vi "FGV_Stop_Error.vi"(7 "Action":enum16{"Read", "Write"}(ring), 8 "Error In (no error)":errorcluster, 10 "Var In":bool) -> (0 "Error Out":errorcluster, 2 "Var Out":bool)   [LabVIEW 2018]
doc: "FGV for stop loop value."
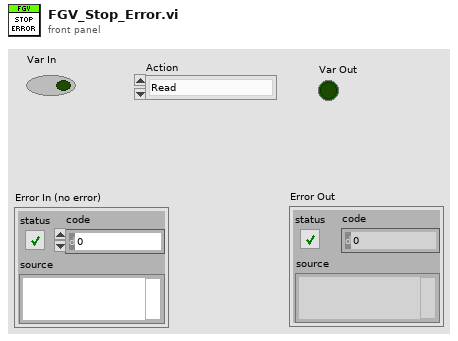
[diagram p1: front panel]
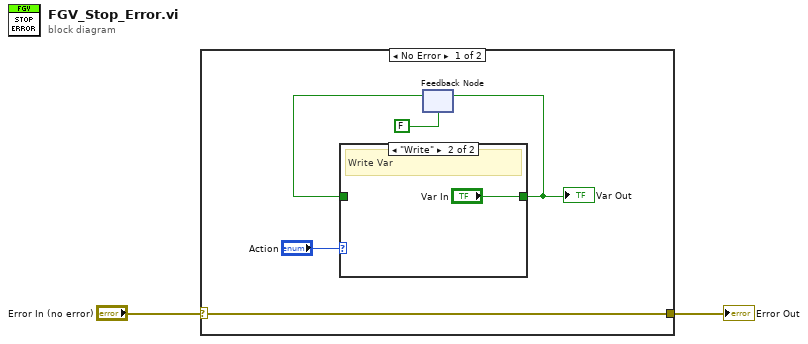
[diagram p0: block diagram]
diagram:
  n1 = case shown="No Error" "Error In (no error)" {
    selector: "Error In (no error)" -> [w3 w10]
    tunnel: [w3 w10] -> w1
    frame No Error {
      n2 = feedback #1(FALSE ("Var In")) -> (w5:bool)
      n3 = case shown="\"Write\"" "Action" {
        tunnel: [w8 "Var In"] -> w6
        tunnel: w5 -> [w8 _]
        frame "Read", Default {
        }
        frame "Write" {
          # "Write Var"
        }
      }
      "Var Out" <- w6
      n4 = feedback-in #1(w6) -> ()
    }
    frame Error {
    }
  }
  "Error Out" <- w1
